vi "Timed Message-Core_Construct.vi"(0 "Initialization Sequence":string, 5 "FTW Actor Instance Configuration":string, 11 "error in (no error)":errorcluster) -> (4 "Timed Message-Core out":refnum<class "Timed Message-Core.lvclass">, 6 "Incoming Requests":refnum<event-registration>, 15 "error out":errorcluster)   [LabVIEW 2012, in "Timed Message-Core.lvclass"]
uses:
  Timed Message-Core.lvclass
  src/Message/Request/FTW-Message-IncomingRequest.lvclass
  Timed Message-Core.lvclass/Timed Message-Core.ctl
  Core/src/Reflection/FTW-Reflection-Type.vi
  Core/src/JSON/FTW-JSON-Core-LibraryFilepath.vi
  Core/src/JSON/FTW-JSON-Core-GetFlattenedValue.vi
  Core/src/JSON/FTW-JSON-Core-LibraryError.vi
  Core/utils/CodeGen/JSON Deserialize/FTW-JSON-Deserialize.xnode
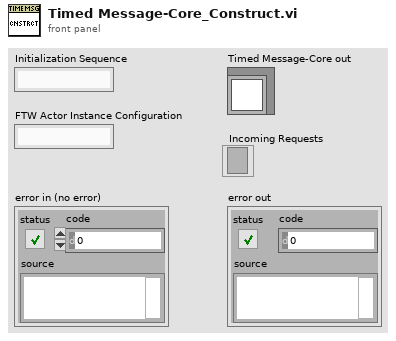
[diagram p1: front panel]
types:
  T1 = cluster{"Message":string, "Address":string, "Interval":i32}
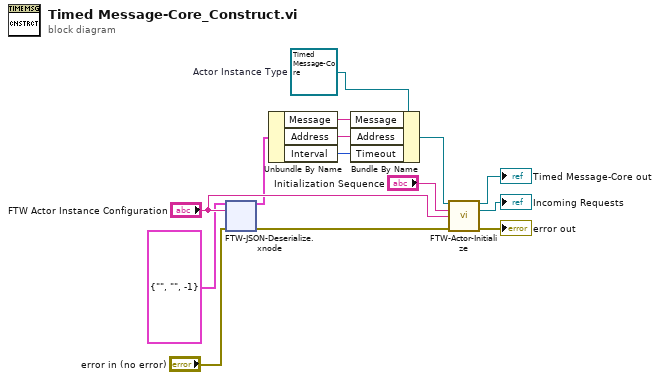
[diagram p0: block diagram]
diagram:
  w12 = refnum<class "Timed Message-Core.lvclass"> refnum  # Actor Instance Type
  n1 = xnode "FTW-JSON-Deserialize.xnode"("Type and Defaults"=T1 {"Message"="", "Address"="", "Interval"=-1}, "JSON String"="FTW Actor Instance Configuration", "error in"="error in (no error)") -> ("Values"=w5:T1, "error out"=w8:errorcluster)
  n2 = Unbundle By Name(w5) -> ("Message"=w3:string, "Address"=w1:string, "Interval"=w2:i32)
  n3 = Bundle By Name(cluster=w12, "Message"=w3, "Address"=w1, "Timeout"=w2) -> (w4:refnum<class "Timed Message-Core.lvclass">)
  n4 = call-dynamic "FTW-Actor-Initialize.vi"("FTW Actor Instance Type"=w4, "Initialization Job Sequence"="Initialization Sequence", "Actor Instance Configuration"="FTW Actor Instance Configuration", "error in"=w8) -> ("FTW Actor Instance"=→"Timed Message-Core out":refnum<class "Timed Message-Core.lvclass">, "Incoming Requests"=→"Incoming Requests":refnum<event-registration>, "error out"=→"error out":errorcluster)  [unwired: 9 in]
